vi "Meas - Meas VI names memory.vi"(7 "Operation":T1=enum."WRITE", 8 "Error In":errorcluster, 11 "Name In":string) -> (0 "Error Out":errorcluster, 3 "Names Out":string[](array[string]))   [LabVIEW 2011]
uses:
  Controls/INIT- READ - WRITE.ctl
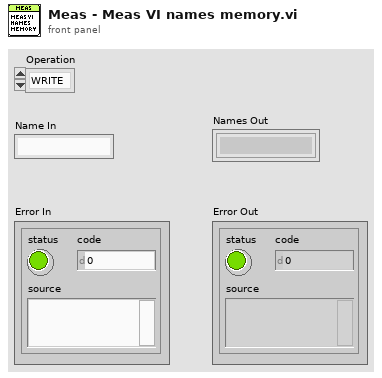
[diagram p1: front panel]
types:
  T1 = typedef "INIT- READ - WRITE.ctl" = enum16{"INIT", "READ", "WRITE"}
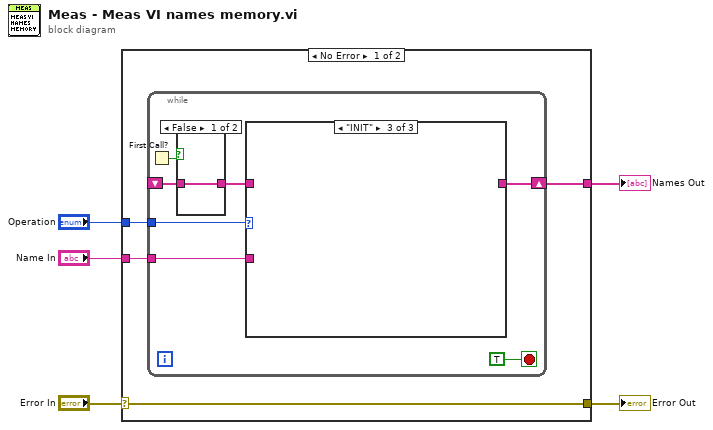
[diagram p0: block diagram]
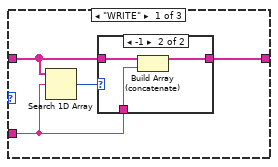
[diagram p3: hidden frame]
diagram:
  n1 = case shown="No Error" "Error In" {
    selector: "Error In" -> [w6 w27]
    tunnel: "Operation" -> [w9 _]
    tunnel: "Name In" -> [w8 _]
    tunnel: [w7 _] -> w3
    tunnel: [w6 w27] -> w1
    frame No Error {
      n2 = while {
        tunnel: w9 -> [w16]
        shift-right: [w14] -> w7
        shift-left: _ -> [w12]
        tunnel: w8 -> [w15]
        stop <- TRUE stop-if-true
        n3 = First Call?() -> (First Call?: T/F=w10:bool)
        n4 = case shown="False" w10 {
          tunnel: w12 -> [w17 _]
          tunnel: [w17 _] -> w11
          frame False {
          }
          frame True {
          }
        }
        n5 = case shown="\"INIT\"" w16 {
          tunnel: w15 -> [w18 _ _]
          tunnel: [w21 w26 _] -> w14
          tunnel: w11 -> [w20 w26 _]
          frame "WRITE" {
            n6 = Search 1D Array(1D array=w20, element=w18) -> (index of element=w19:i32)  [unwired: 1 in]
            n7 = case shown="-1" w19 {
              tunnel: w18 -> [_ w25]
              tunnel: [w22 w24] -> w21
              tunnel: w20 -> [w22 w23]
              frame Default {
              }
              frame -1 {
                n8 = Build Array (concatenate)(w23, w25) -> (w24:string[])
              }
            }
          }
          frame "READ" {
          }
          frame "INIT" {
          }
        }
      }
    }
    frame Error {
    }
  }
  "Names Out" <- w3
  "Error Out" <- w1
